vi "GetLeftPeakAndRightPeakvi.vi"(0 "Peak position":dbl, 1 "Connection Cluster in":T1, 5 "Target thickness":dbl, 11 "Thickness tolerance":dbl) -> (3 "Connection Cluster out":T1, 4 "Peak detected? left":bool, 6 "Peak (left)":dbl, 10 "Peak detected? right":bool, 15 "Peak (right)":dbl)   [LabVIEW 2013]
uses:
  Global.vi
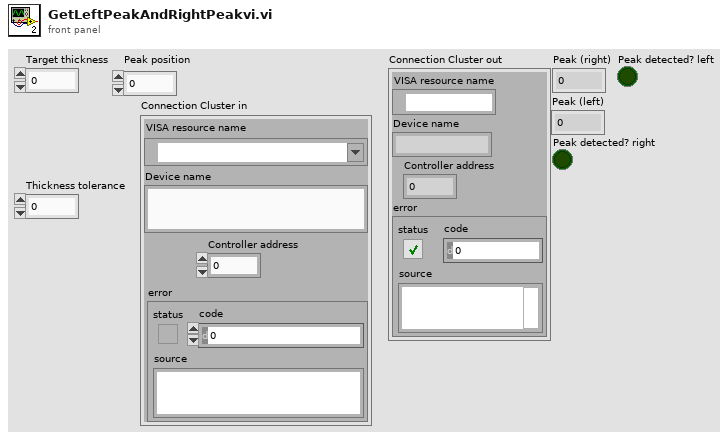
[diagram p1: front panel]
types:
  T1 = cluster{"VISA resource name":refnum<visa-resource-name>, "Device name":string, "Controller address":i32, "error":errorcluster}
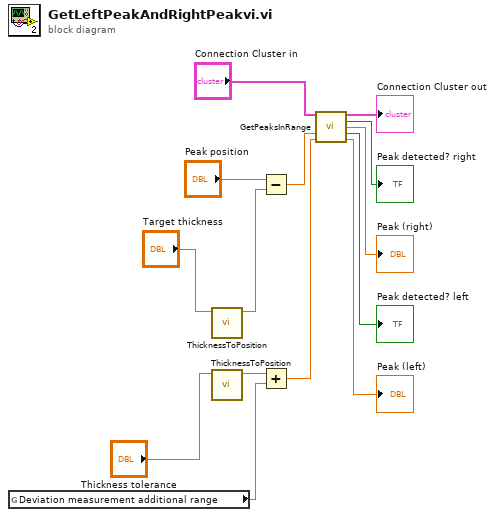
[diagram p0: block diagram]
diagram:
  n1 = global read "Global.vi" "Deviation measurement additional range"() -> (w7:dbl)
  n2 = call "ThicknessToPosition.vi"("Thickness"="Target thickness") -> ("Position"=w13:dbl)  [unwired: 10 in]
  n3 = call "ThicknessToPosition.vi"("Thickness"="Thickness tolerance") -> ("Position"=w8:dbl)  [unwired: 10 in]
  n4 = Subtract(x="Peak position", y=w13) -> (x-y=w10:dbl)
  n5 = Add(x=w8, y=w7) -> (x+y=w6:dbl)
  n6 = call "GetPeaksInRange.vi"("Connection Cluster in"="Connection Cluster in", "Start Position"=w10, "Fine range"=w6) -> ("Connection Cluster out"=→"Connection Cluster out":T1, "Peak detected? right"=→"Peak detected? right":bool, "Peak (right)"=→"Peak (right)":dbl, "Peak detected? left"=→"Peak detected? left":bool, "Peak (left)"=→"Peak (left)":dbl)  [unwired: 8 in]
